vi "Main Analysis-Incomplete.vi"(0 "selected path":path, 5 "VI reference":refnum<vi>, 11 "Error In":errorcluster) -> (2 "Resistance (Out)":dbl, 3 "error?":bool, 4 "Filename Out":path=path "E:/LabVIEW/Data/Test Data/Subj-Austin_Trial-1_Condition-None.lvm" caption="Filename", 6 "SGP":dbl, 8 "SPL":dbl format="%0.3f", 10 "PTP":dbl, 13 "Start Flow":dbl format="%0.3f", 14 "End Flow":dbl format="%0.3f", 15 "Error Out":errorcluster)   [LabVIEW 2020]
panel:
  # "Don't worry about this front panel.  It never gets displayed."
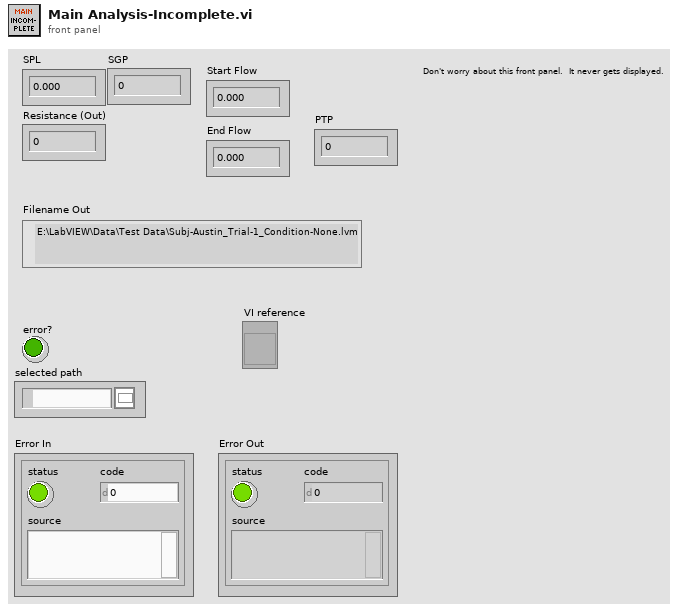
[diagram p1: front panel]
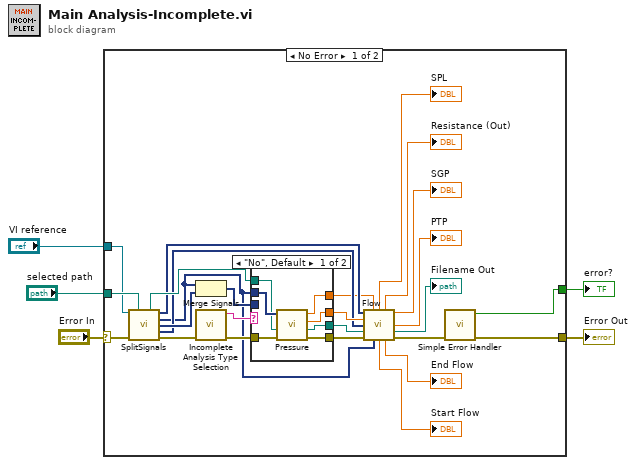
[diagram p0: block diagram]
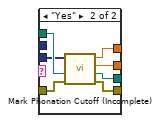
[diagram p2: hidden frame]
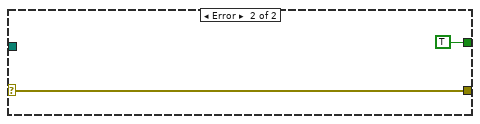
[diagram p3: hidden frame]
diagram:
  n1 = case shown="No Error" "Error In" {
    selector: "Error In" -> [w31 w47]
    tunnel: "selected path" -> [w30 _]
    tunnel: [w29 w47] -> w3
    tunnel: [w28 TRUE ("error?")] -> w2
    tunnel: "VI reference" -> [w6 _]
    frame No Error {
      n2 = call "SplitSignals.vi"("VI reference"=w6, "Filename"=w30, "Error In"=w31) -> ("Filename Out"=w22:path, "Flow"=w20:dynamicdata, "Pressure"=w7:dynamicdata, "Audio"=w24:dynamicdata, "SPL"=w17:dynamicdata, "Error Out"=w27:errorcluster)  [unwired: 5 in, 2 out]
      n3 = Merge Signals(w7, w24) -> (w23:dynamicdata)
      n4 = call "Incomplete Analysis Type Selection.vi"("Error In"=w27) -> ("Error Out"=w25:errorcluster, "Yes or No"=w26:string)  [unwired: 9 in]
      n5 = case shown="\"No\", Default" w26 {
        tunnel: w25 -> [w38 w45]
        tunnel: [w37 w44] -> w21
        tunnel: w23 -> [_ w42]
        tunnel: w22 -> [w33 w43]
        tunnel: w7 -> [w36 _]
        tunnel: [w35 w41] -> w19
        tunnel: [w34 w40] -> w18
        tunnel: [w32 w39] -> w9
        frame "No", Default {
          n6 = call "Pressure.vi"("Error In"=w38, "File Path"=w33, "Pressure"=w36) -> ("Error Out"=w37:errorcluster, "File Path Indicator"=w34:path, "Interruption Time"=w35:dbl, "Pressure"=w32:dbl)  [unwired: 4 in]
        }
        frame "Yes" {
          n7 = call "Mark Phonation Cutoff (Incomplete).vi"("Error In"=w45, "File Path"=w43, "Pressure/Audio"=w42) -> ("Error Out"=w44:errorcluster, "File Path Indicator"=w40:path, "Interruption Time"=w41:dbl, "Cutoff Pressure"=w39:dbl)  [unwired: 4 in]
        }
      }
      n8 = call "Flow.vi"("Flow"=w20, "Cuttoff Pressure"=w9, "Interruption Time"=w19, "SPL"=w17, "File Name In"=w18, "Error In"=w21, "Pressure"=w7) -> ("SPL"=→"SPL":dbl, "Resistance (Out)"=→"Resistance (Out)":dbl, "SGP"=→"SGP":dbl, "PTP"=→"PTP":dbl, "File Name"=→"Filename Out":path, "Start Flow"=→"Start Flow":dbl, "End Flow"=→"End Flow":dbl, "Error Out"=w16:errorcluster)  [unwired: 1 out]
      n9 = call <vilib>:"Simple Error Handler.vi"("error in (no error)"=w16) -> ("error?"=w28:bool, "error out"=w29:errorcluster)  [unwired: 4 in, 3 out]
    }
    frame Error {
    }
  }
  "Error Out" <- w3
  "error?" <- w2
